vi "Set_magnetrons_to_standby.vi"(1 "error in":errorcluster, 2 "Data in":T1) -> (0 "error out":errorcluster)   [LabVIEW 2015, in "Steps.lvlib"]
uses:
  Steps.lvlib
  Type_Defs/Data.ctl
  Type_Defs/Diagnostics.ctl
  Type_Defs/Systems.ctl
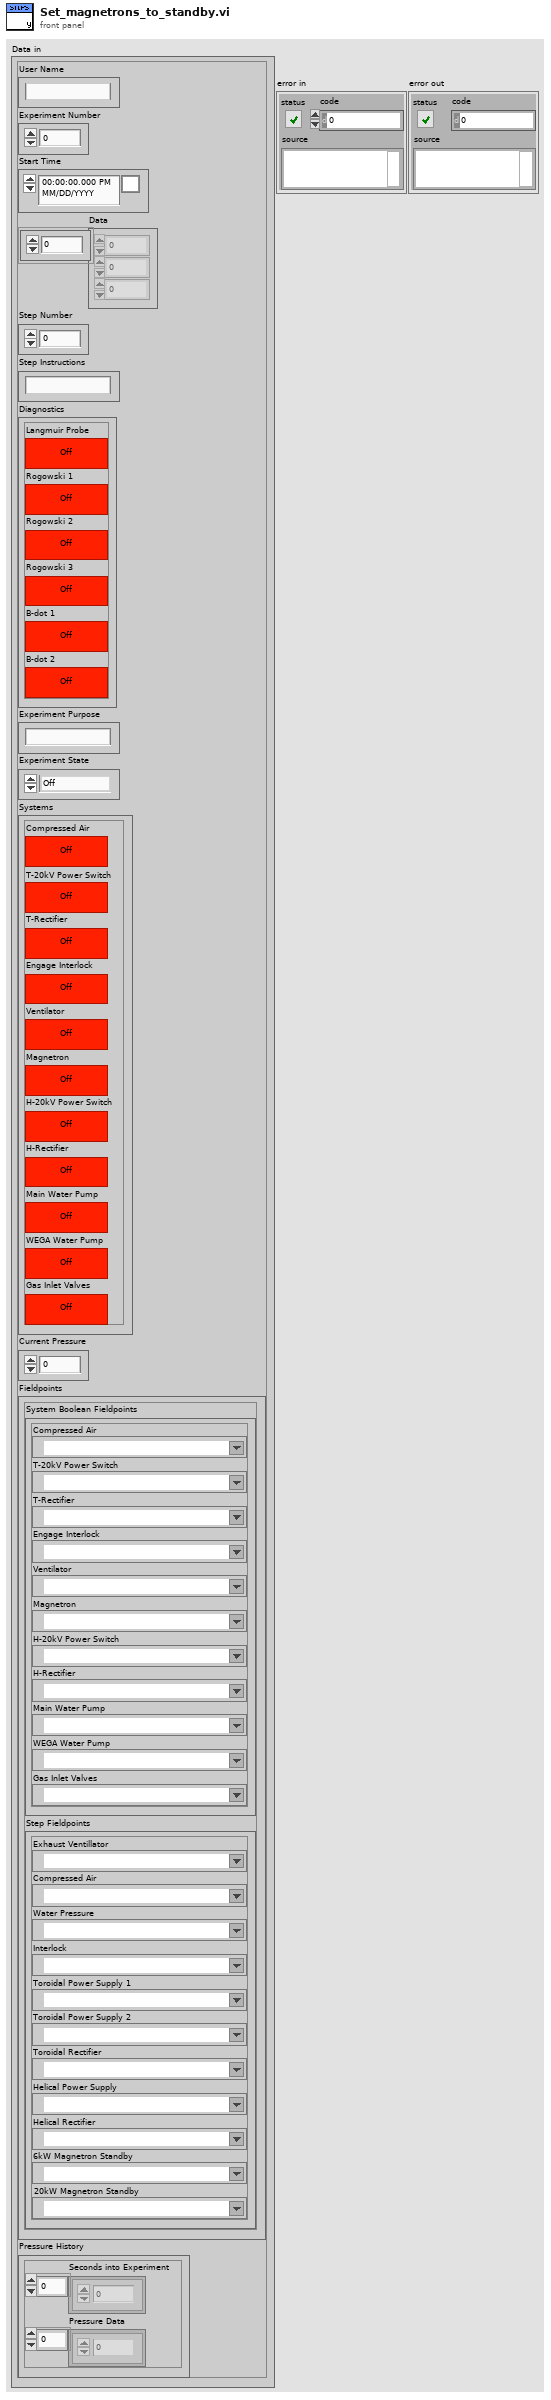
[diagram p1: front panel]
types:
  T1 = typedef "Data.ctl" = cluster{"User Name":string, "Experiment Number":i32, "Start Time":timestamp, "Data":dbl[], "Step Number":i32, "Step Instructions":string, "Diagnostics":T2, "Experiment Purpose":string, "Experiment State":enum16{"Off", "Setting Up", "Ready", "In Progress", "Shutting Down"}, "Systems":T3, "Current Pressure":dbl, "Fieldpoints":cluster{"System Boolean Fieldpoints":cluster{"Compressed Air":refnum<k21>, "T-20kV Power Switch":refnum<k21>, "T-Rectifier":refnum<k21>, "Engage Interlock":refnum<k21>, "Ventilator":refnum<k21>, "Magnetron":refnum<k21>, "H-20kV Power Switch":refnum<k21>, "H-Rectifier":refnum<k21>, "Main Water Pump":refnum<k21>, "WEGA Water Pump":refnum<k21>, "Gas Inlet Valves":refnum<k21>}, "Step Fieldpoints":cluster{"Exhaust Ventillator":refnum<k21>, "Compressed Air":refnum<k21>, "Water Pressure":refnum<k21>, "Interlock":refnum<k21>, "Toroidal Power Supply 1":refnum<k21>, "Toroidal Power Supply 2":refnum<k21>, "Toroidal Rectifier":refnum<k21>, "Helical Power Supply":refnum<k21>, "Helical Rectifier":refnum<k21>, "6kW Magnetron Standby":refnum<k21>, "20kW Magnetron Standby":refnum<k21>}}, "Pressure History":cluster{"Seconds into Experiment":i32[], "Pressure Data":dbl[]}}
  T2 = typedef "Diagnostics.ctl" = cluster{"Langmuir Probe":bool, "Rogowski 1":bool, "Rogowski 2":bool, "Rogowski 3":bool, "B-dot 1":bool, "B-dot 2":bool}
  T3 = typedef "Systems.ctl" = cluster{"Compressed Air":bool, "T-20kV Power Switch":bool, "T-Rectifier":bool, "Engage Interlock":bool, "Ventilator":bool, "Magnetron":bool, "H-20kV Power Switch":bool, "H-Rectifier":bool, "Main Water Pump":bool, "WEGA Water Pump":bool, "Gas Inlet Valves":bool}
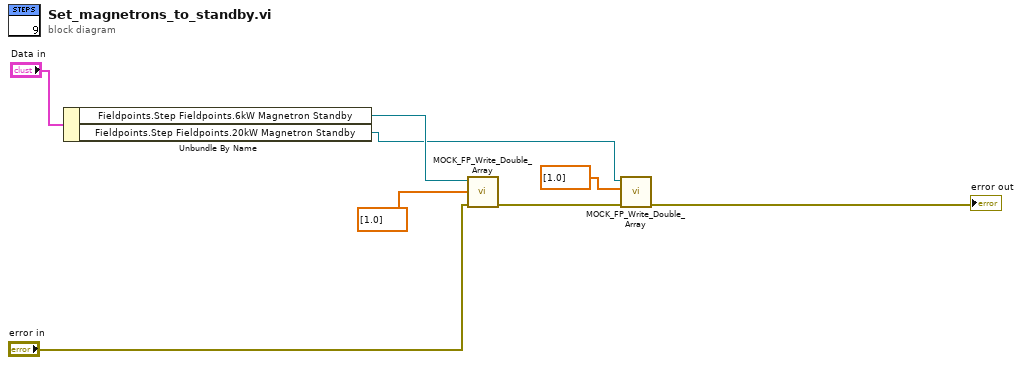
[diagram p0: block diagram]
diagram:
  n1 = Unbundle By Name("Data in") -> ("Fieldpoints.Step Fieldpoints.6kW Magnetron Standby"=w5:refnum<k21>, "Fieldpoints.Step Fieldpoints.20kW Magnetron Standby"=w2:refnum<k21>)
  n2 = call "MOCK_FP_Write_Double_Array.vi"("error in"="error in", "values"=dbl[] [1.0], "FieldPoint IO Point In"=w5) -> ("error out"=w4:errorcluster)  [unwired: 6 in, 2 out]
  n3 = call "MOCK_FP_Write_Double_Array.vi"("error in"=w4, "values"=dbl[] [1.0], "FieldPoint IO Point In"=w2) -> ("error out"=→"error out":errorcluster)  [unwired: 6 in, 2 out]
